vi "Parse MKS Pressure String.vi"(8 "error in (no error)":errorcluster, 11 "String":string) -> (0 "error out":errorcluster, 3 "Pressure 1":dbl)   [LabVIEW 2020, in "MKS_PressureTransducer.lvclass"]
uses:
  MKS_PressureTransducer.lvclass
panel:
  out "substring":string
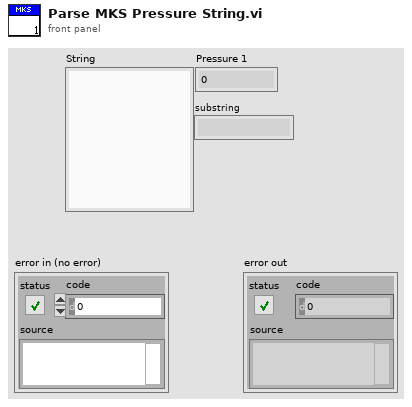
[diagram p1: front panel]
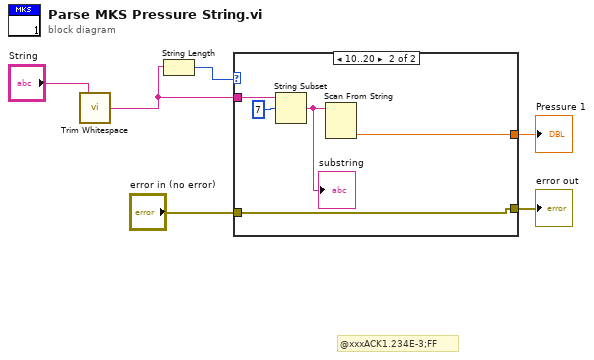
[diagram p0: block diagram]
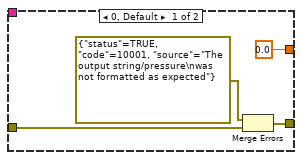
[diagram p2: hidden frame]
diagram:
  # "@xxxACK1.234E-3;FF"
  n1 = call "Trim Whitespace.vi"("string"="String") -> ("trimmed string"=w1:string)  [unwired: 1 in]
  n2 = String Length(string=w1) -> (length=w6:i32)
  n3 = case shown="10..20" w6 {
    tunnel: w1 -> [_ w15]
    tunnel: "error in (no error)" -> [w10 w12]
    tunnel: [w9 w12] -> w4
    tunnel: [0.0 w11] -> w3
    frame 0, Default {
      n4 = Merge Errors(errorcluster {"status"=TRUE, "code"=10001, "source"="The output string/pressure\nwas not formatted as expected"} ("error in (no error)"), w10) -> (w9:errorcluster)
    }
    frame 10..20 {
      n5 = String Subset(string=w15, offset (0)=7) -> (substring=w13:string)  [unwired: 1 in]
      "substring" <- w13
      n6 = Scan From String(input string=w13) -> (output 1=w11:dbl)  [unwired: 4 in, 3 out]
    }
  }
  "error out" <- w4
  "Pressure 1" <- w3
